vi "Convert Data to Gain values.vi"(0 "Messages":T1(array[cluster])) -> (14 "Gain A":sgl, 15 "Gain B":sgl, 16 "Gain C":sgl, 17 "Gain D":sgl, 18 "Gain E":sgl, 19 "Gain F":sgl)   [LabVIEW 2025]
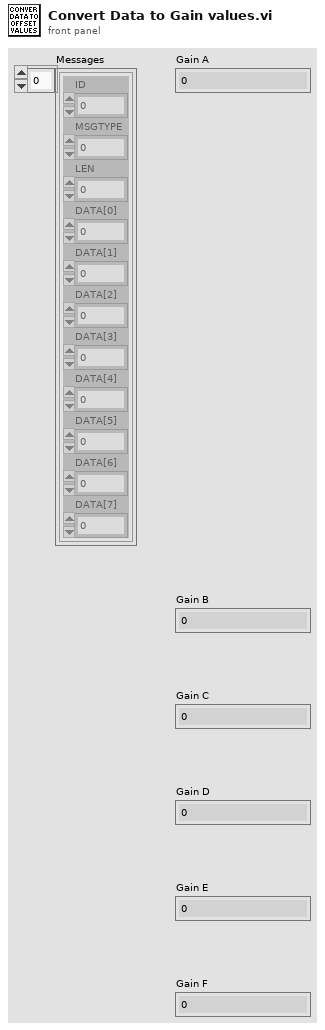
[diagram p1: front panel]
types:
  T1 = cluster{"ID":u32, "MSGTYPE":u8, "LEN":u8, "DATA[0]":u8, "DATA[1]":u8, "DATA[2]":u8, "DATA[3]":u8, "DATA[4]":u8, "DATA[5]":u8, "DATA[6]":u8, "DATA[7]":u8}[]
  T2 = cluster{"ID":u32, "MSGTYPE":u8, "LEN":u8, "DATA[0]":u8, "DATA[1]":u8, "DATA[2]":u8, "DATA[3]":u8, "DATA[4]":u8, "DATA[5]":u8, "DATA[6]":u8, "DATA[7]":u8}
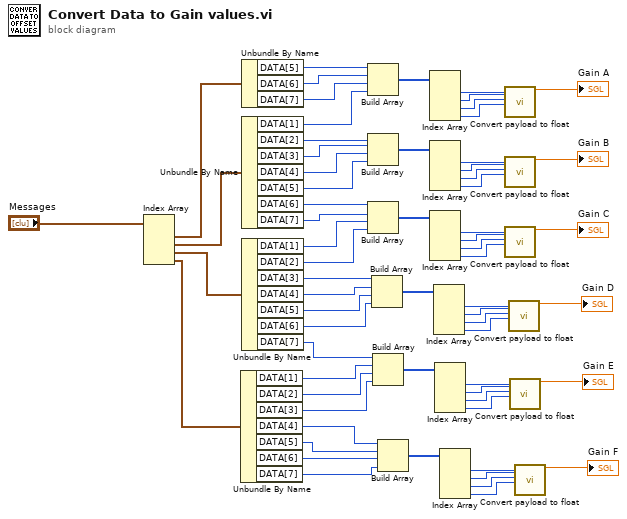
[diagram p0: block diagram]
diagram:
  n1 = Index Array(array="Messages") -> (element #1=w64:T2, element #2=w63:T2, element #3=w62:T2, element #4=w1:T2)  [unwired: 4 in]
  n2 = Unbundle By Name(w1) -> ("DATA[1]"=w14:u8, "DATA[2]"=w13:u8, "DATA[3]"=w12:u8, "DATA[4]"=w5:u8, "DATA[5]"=w4:u8, "DATA[6]"=w3:u8, "DATA[7]"=w2:u8)
  n3 = Unbundle By Name(w64) -> ("DATA[5]"=w61:u8, "DATA[6]"=w60:u8, "DATA[7]"=w59:u8)
  n4 = Unbundle By Name(w63) -> ("DATA[1]"=w58:u8, "DATA[2]"=w57:u8, "DATA[3]"=w56:u8, "DATA[4]"=w55:u8, "DATA[5]"=w54:u8, "DATA[6]"=w53:u8, "DATA[7]"=w52:u8)
  n5 = Unbundle By Name(w62) -> ("DATA[1]"=w51:u8, "DATA[2]"=w50:u8, "DATA[3]"=w25:u8, "DATA[4]"=w24:u8, "DATA[5]"=w23:u8, "DATA[6]"=w22:u8, "DATA[7]"=w15:u8)
  n6 = Build Array(w61, w60, w59, w58) -> (w49:u8[])
  n7 = Build Array(w57, w56, w55, w54) -> (w39:u8[])
  n8 = Build Array(w53, w52, w51, w50) -> (w34:u8[])
  n9 = Build Array(w25, w24, w23, w22) -> (w30:u8[])
  n10 = Build Array(w15, w14, w13, w12) -> (w17:u8[])
  n11 = Build Array(w5, w4, w3, w2) -> (w10:u8[])
  n12 = Index Array(array=w49) -> (element #1=w48:u8, element #2=w47:u8, element #3=w46:u8, element #4=w45:u8)  [unwired: 4 in]
  n13 = Index Array(array=w39) -> (element #1=w40:u8, element #2=w41:u8, element #3=w42:u8, element #4=w43:u8)  [unwired: 4 in]
  n14 = Index Array(array=w34) -> (element #1=w38:u8, element #2=w37:u8, element #3=w36:u8, element #4=w35:u8)  [unwired: 4 in]
  n15 = Index Array(array=w30) -> (element #1=w26:u8, element #2=w27:u8, element #3=w28:u8, element #4=w29:u8)  [unwired: 4 in]
  n16 = Index Array(array=w17) -> (element #1=w21:u8, element #2=w20:u8, element #3=w19:u8, element #4=w18:u8)  [unwired: 4 in]
  n17 = Index Array(array=w10) -> (element #1=w6:u8, element #2=w7:u8, element #3=w8:u8, element #4=w9:u8)  [unwired: 4 in]
  n18 = call "Convert payload to float.vi"("Byte1"=w48, "Byte2"=w47, "Byte3"=w46, "Byte4"=w45) -> ("FloatNumber"=→"Gain A":sgl)  [unwired: 15 in]
  n19 = call "Convert payload to float.vi"("Byte1"=w40, "Byte2"=w41, "Byte3"=w42, "Byte4"=w43) -> ("FloatNumber"=→"Gain B":sgl)  [unwired: 15 in]
  n20 = call "Convert payload to float.vi"("Byte1"=w38, "Byte2"=w37, "Byte3"=w36, "Byte4"=w35) -> ("FloatNumber"=→"Gain C":sgl)  [unwired: 15 in]
  n21 = call "Convert payload to float.vi"("Byte1"=w26, "Byte2"=w27, "Byte3"=w28, "Byte4"=w29) -> ("FloatNumber"=→"Gain D":sgl)  [unwired: 15 in]
  n22 = call "Convert payload to float.vi"("Byte1"=w21, "Byte2"=w20, "Byte3"=w19, "Byte4"=w18) -> ("FloatNumber"=→"Gain E":sgl)  [unwired: 15 in]
  n23 = call "Convert payload to float.vi"("Byte1"=w6, "Byte2"=w7, "Byte3"=w8, "Byte4"=w9) -> ("FloatNumber"=→"Gain F":sgl)  [unwired: 15 in]
